vi "Test App Adding Second Process and Starting App Again.vi"(8 "error in (no error)":errorcluster, 11 "Application Test In":refnum<class "Application Dev Test.lvclass">) -> (0 "error out":errorcluster, 3 "Application Test Out":refnum<class "Application Dev Test.lvclass">)   [LabVIEW 2020, in "Application Dev Test.lvclass"]
uses:
  Application Dev Test.lvclass
  C:/Program Files (x86)/National Instruments/LabVIEW 2020/vi.lib/Astemes/LUnit/Test Case.lvclass
  source/Framework Test Suite/Mock Process/Mock Process.lvclass
  C:/Git/astemes-triarc-framework/source/Framework/Process/Process.lvclass
  source/Framework/Process/Process.lvclass/Process.ctl
  source/Framework/Application/Application.lvclass/Application.ctl
  <vilib>/Astemes/LUnit/Test Case.lvclass/Test Case.ctl
  <vilib>/Astemes/LUnit/LUnit Assertion Result.lvclass/LUnit Assertion Result.ctl
  <vilib>/Astemes/LUnit/LUnit Test Case Result.lvclass/LUnit Test Case Result.ctl
  <vilib>/Astemes/LUnit/LUnit Method Result.lvclass/LUnit Method Result.ctl
  source/Framework/Application/Private/Add Process to Map.vi
  source/Framework/Application/Private/Start Idle Processes if Running.vi
  source/Framework/Application/Private/Throw Error If Process Already in App.vi
  source/Framework/Process/Protected/Messaging/Enqueue Message.vi
  source/Framework/Process/Public/Lifecycle/Get Lifecycle State.vi
  source/Framework/Process/Protected/SubVIs/Set Context.vi
  source/Framework/Process/Private/SubVIs/Wait for finish.vi
  source/Framework/Process/Private/SubVIs/Set Lifecycle State.vi
  <vilib>/Astemes/LUnit/Palette/Fail.vi
  <vilib>/Astemes/LUnit/Palette/Pass.vi
  <vilib>/Astemes/LUnit/Set Assertion Type.vi
  source/Framework/Application/Public/Get Process.vi
  source/Framework/Process/Private/SubVIs/Handle Debug Data.vi
  <vilib>/Utility/error.llb/Clear Errors.vi
  source/Framework/Process/Public/Lifecycle/Leave Process Loop.vi
  <vilib>/Astemes/LUnit/Add test result.vi
  <vilib>/Astemes/LUnit/LUnit Write Passed.vi
  <vilib>/Astemes/LUnit/LUnit Write Message.vi
  <vilib>/Astemes/LUnit/LUnit Write Description.vi
  <vilib>/Astemes/LUnit/LUnit Write Assertion Type.vi
  source/Framework/Application/Private/Retrieve Process from App.vi
  source/Framework/Application/Private/Parse Process Name.vi
  source/Framework/Application/Private/Get Process from Map.vi
  source/Framework/Logging/Log Debug.vi
  <vilib>/AdvancedString/1D String Array to Delimited String.vi
  <vilib>/Utility/High Resolution Relative Seconds.vi
  <vilib>/Astemes/LUnit/LUnit Record Assertion Result.vi
  source/Framework/Process/Protected/Messaging/Request Message.vi
  <vilib>/AdvancedString/Delimited String to 1D String Array.vi
  <vilib>/Astemes/LUnit/LUnit Aggregate Assertion Results.vi
  source/Framework/Process/Private/SubVIs/Enqueue Request Message.vi
  <vilib>/Astemes/LUnit/Assertion Result/LUnit Read Status.vi
  <vilib>/Astemes/LUnit/LUnit Read Message.vi
  <vilib>/Astemes/LUnit/LUnit Read Description.vi
  <vilib>/Astemes/LUnit/Method Result/LUnit Merge Status.vi
  <vilib>/Astemes/LUnit/LUnit Concatenate result strings.vi
  source/Framework/Application/Application.lvclass
  <vilib>/Utility/error.llb/Error Cluster From Error Code.vi
  source/Framework/Process/Public/Read Name.vi
  source/Framework/Process/Private/SubVIs/Wait for Response Message.vi
  source/Framework/Process/Process.lvclass
  <vilib>/Astemes/LUnit/LUnit Assertion Result.lvclass
  Application Dev Test.lvclass/Application Dev Test.ctl
  <vilib>/Astemes/LUnit/Test Case.lvclass
panel:
  out "Messages 2":string[](array[string])
  out "Messages":string[](array[string])
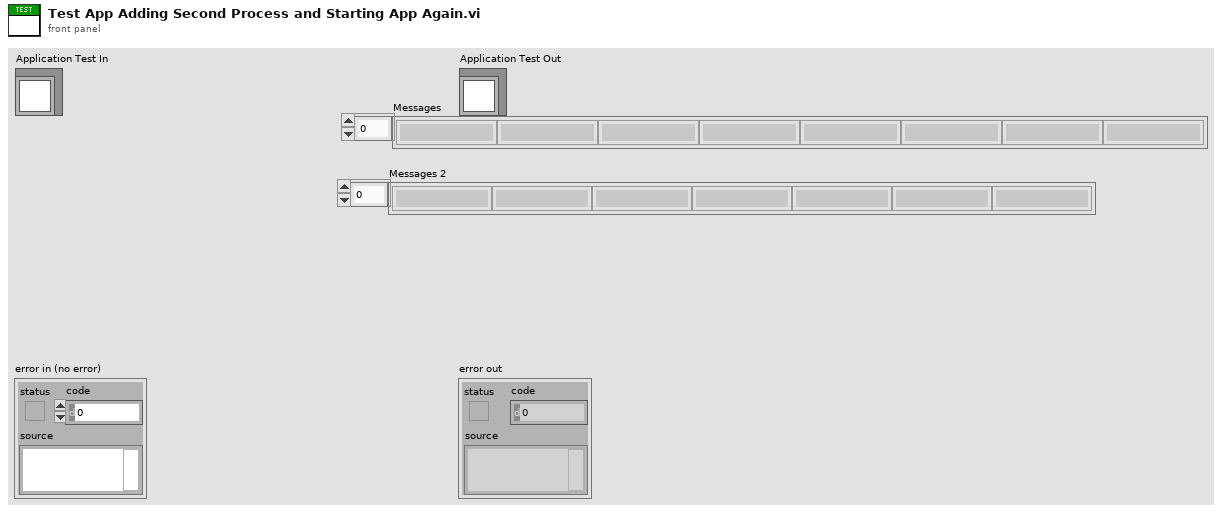
[diagram p1: front panel]
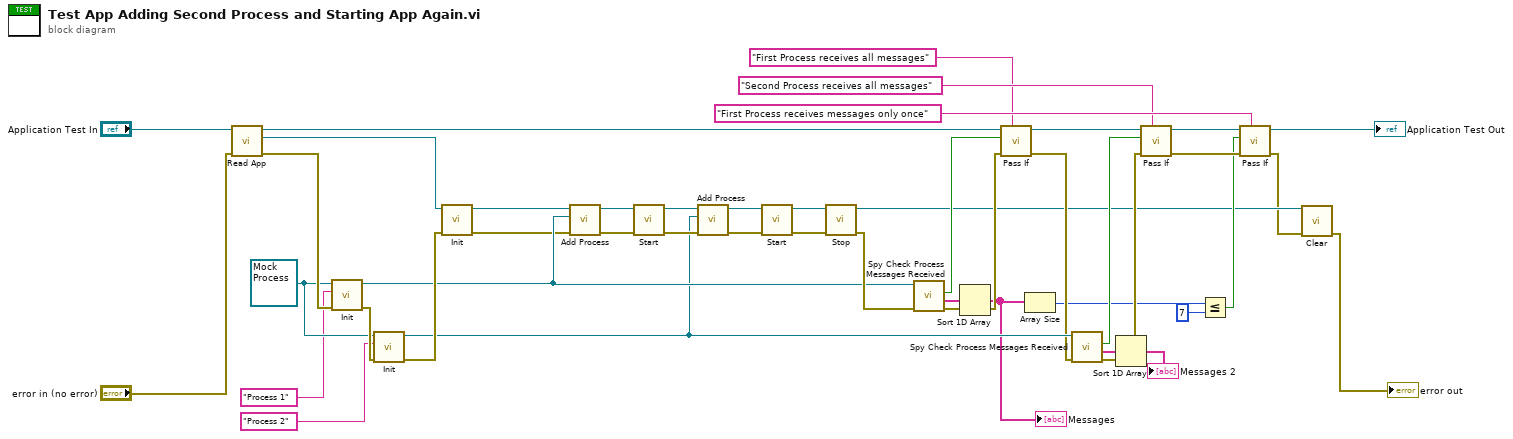
[diagram p0: block diagram]
diagram:
  w31 = refnum<class "Mock Process.lvclass"> refnum ("Mock Classes.lvlib:Mock Process.lvclass")
  n1 = call "Read App.vi"("error in (no error)"="error in (no error)", "Application Test In"="Application Test In") -> ("error out"=w34:errorcluster, "App out"=w35:refnum<class "Application.lvclass">, "Application Test Out"=w44:refnum<class "Application Dev Test.lvclass">)  [unwired: 7 in]
  n2 = call-dynamic "Init.vi"("error in (no error)"=w34, "Name"="Process 1", "Mock Process In"=w31) -> ("error out"=w40:errorcluster, "Mock Process Out"=w38:refnum<class "Mock Process.lvclass">)  [unwired: 7 in]
  n3 = call-dynamic "Init.vi"("error in (no error)"=w40, "Name"="Process 2", "Mock Process In"=w31) -> ("error out"=w39:errorcluster, "Mock Process Out"=w26:refnum<class "Mock Process.lvclass">)  [unwired: 7 in]
  n4 = call-dynamic "Init.vi"("error in (no error)"=w39, "Process In"=w35) -> ("error out"=w9:errorcluster, "Process Out"=w42:refnum<class "Application.lvclass">)  [unwired: 8 in]
  n5 = call "Add Process.vi"("error in (no error)"=w9, "Process"=w38, "Application In"=w42) -> ("error out"=w27:errorcluster, "Application Out"=w30:refnum<class "Application.lvclass">)  [unwired: 7 in]
  n6 = call "Start.vi"("error in (no error)"=w27, "Process In"=w30) -> ("error out"=w28:errorcluster, "Process Out"=w29:refnum<class "Application.lvclass">)  [unwired: 7 in, 1 out]
  n7 = call "Add Process.vi"("error in (no error)"=w28, "Process"=w26, "Application In"=w29) -> ("error out"=w36:errorcluster, "Application Out"=w37:refnum<class "Application.lvclass">)  [unwired: 7 in]
  n8 = call "Start.vi"("error in (no error)"=w36, "Process In"=w37) -> ("error out"=w32:errorcluster, "Process Out"=w33:refnum<class "Application.lvclass">)  [unwired: 7 in, 1 out]
  n9 = call "Stop.vi"("error in (no error)"=w32, "Process In"=w33) -> ("error out"=w41:errorcluster, "Process Out"=w3:refnum<class "Application.lvclass">)  [unwired: 7 in, 1 out]
  n10 = call "Spy Check Process Messages Received.vi"("error in (no error)"=w41, "Mock Process In"=w38) -> ("error out"=w23:errorcluster, "Messages"=w15:string[], "Messages received?"=w21:bool)  [unwired: 6 in, 1 out]
  n11 = Sort 1D Array(array=w15) -> (sorted array=w7:string[])
  "Messages" <- w7
  n12 = call <vilib>:"Pass If.vi"("Description"="First Process receives all messages", "error in (no error)"=w23, "Pass?"=w21, "LUnit Test Case In"=w44) -> ("error out"=w22:errorcluster, "LUnit Test Case Out"=w25:refnum<class "Application Dev Test.lvclass">)  [unwired: 6 in]
  n13 = Array Size(array=w7) -> (size(s)=w6:i32)
  n14 = call "Spy Check Process Messages Received.vi"("error in (no error)"=w22, "Mock Process In"=w26) -> ("error out"=w18:errorcluster, "Messages"=w17:string[], "Messages received?"=w19:bool)  [unwired: 6 in, 1 out]
  n15 = Sort 1D Array(array=w17) -> (sorted array=→"Messages 2":string[])
  n16 = call <vilib>:"Pass If.vi"("Description"="Second Process receives all messages", "error in (no error)"=w18, "Pass?"=w19, "LUnit Test Case In"=w25) -> ("error out"=w16:errorcluster, "LUnit Test Case Out"=w24:refnum<class "Application Dev Test.lvclass">)  [unwired: 6 in]
  n17 = Less Or Equal?(x=w6, y=7) -> (x <= y?=w4:bool)
  n18 = call <vilib>:"Pass If.vi"("Description"="First Process receives messages only once", "error in (no error)"=w16, "Pass?"=w4, "LUnit Test Case In"=w24) -> ("error out"=w2:errorcluster, "LUnit Test Case Out"=→"Application Test Out":refnum<class "Application Dev Test.lvclass">)  [unwired: 6 in]
  n19 = call-dynamic "Clear.vi"("error in (no error)"=w2, "Application In"=w3) -> ("error out"=→"error out":errorcluster)  [unwired: 9 in]
